vi "Read Trigger.vi"(8 "error in (no error)":errorcluster, 11 "VISA resource name":refnum<visa-resource-name>) -> (0 "error out":errorcluster, 2 "Trigger Value":i32, 3 "VISA resource name out":refnum<visa-resource-name>)   [LabVIEW 2016, in "EFD Ultimus V.lvlib"]
doc: "Reads the 5-digit trigger value of the current memory location.\n\nHost Format: ER--\n\nReturn Format: D0TVttttt\nttttt: 5-Digit trigger value. Range is 00000 to 99999"
uses:
  EFD Ultimus V.lvlib
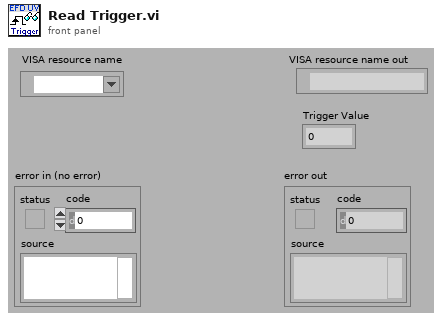
[diagram p1: front panel]
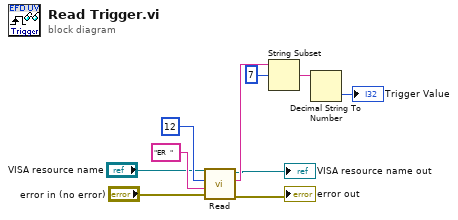
[diagram p0: block diagram]
diagram:
  n1 = call "Read.vi"("error in (no error)"="error in (no error)", "Command To Write"="ER  ", "Bytes to Read (11)"=u32 12 ("Bytes to Read"), "VISA resource name"="VISA resource name") -> ("error out"=→"error out":errorcluster, "Ultimus V Feedback Data"=w8:string, "VISA resource name out"=→"VISA resource name out":refnum<visa-resource-name>)  [unwired: 5 out]
  n2 = String Subset(string=w8, offset (0)=7) -> (substring=w9:string)  [unwired: 1 out]
  n3 = Decimal String To Number(string=w9) -> (number=→"Trigger Value":i32)  [unwired: 3 out]
